vi "Create CAN Tag.vi"(8 "error in (no error)":errorcluster, 11 "CVT Tags to Create":T1) -> (0 "error out":errorcluster, 3 "CVT Tags to Create 2":T1)   [LabVIEW 2016, in "CVT.lvlib"]
uses:
  CVT.lvlib
  <vilib>/NI/Current Value Table/Type Defs/File Format.ctl
  <vilib>/NI/Current Value Table/Type Defs/Single Tag.ctl
  <vilib>/NI/Current Value Table/Type Defs/Data Types.ctl
  <vilib>/NI/Current Value Table/Type Defs/Tag Grouping set.ctl
  <vilib>/NI/Current Value Table/Current Value Table.lvlib
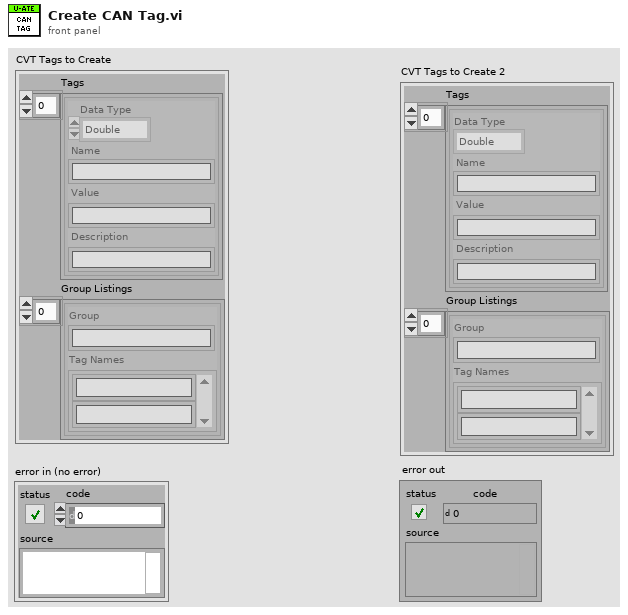
[diagram p1: front panel]
types:
  T1 = typedef "Current Value Table.lvlib/File Format.ctl" = cluster{"Tags":T2[], "Group Listings":T4[]}
  T2 = typedef "Current Value Table.lvlib/Single Tag.ctl" = cluster{"Data Type":T3, "Name":string, "Value":string, "Description":string}
  T3 = typedef "Current Value Table.lvlib/Data Types.ctl" = enum16{"Double", "Single", "I64", "I32", "I16", "I8", "U64", "U32", "U16", "U8", "String", "Boolean", "Array of U8", "Array of U16", "Array of U32", "Array of U64", "Array of I64", "Array of I32", "Array of I16", "Array of I8", "Array of Double", "Array of Single", "Array of Boolean", "Array of String"}
  T4 = typedef "Current Value Table.lvlib/Tag Grouping set.ctl" = cluster{"Group":string, "Tag Names":string[]}
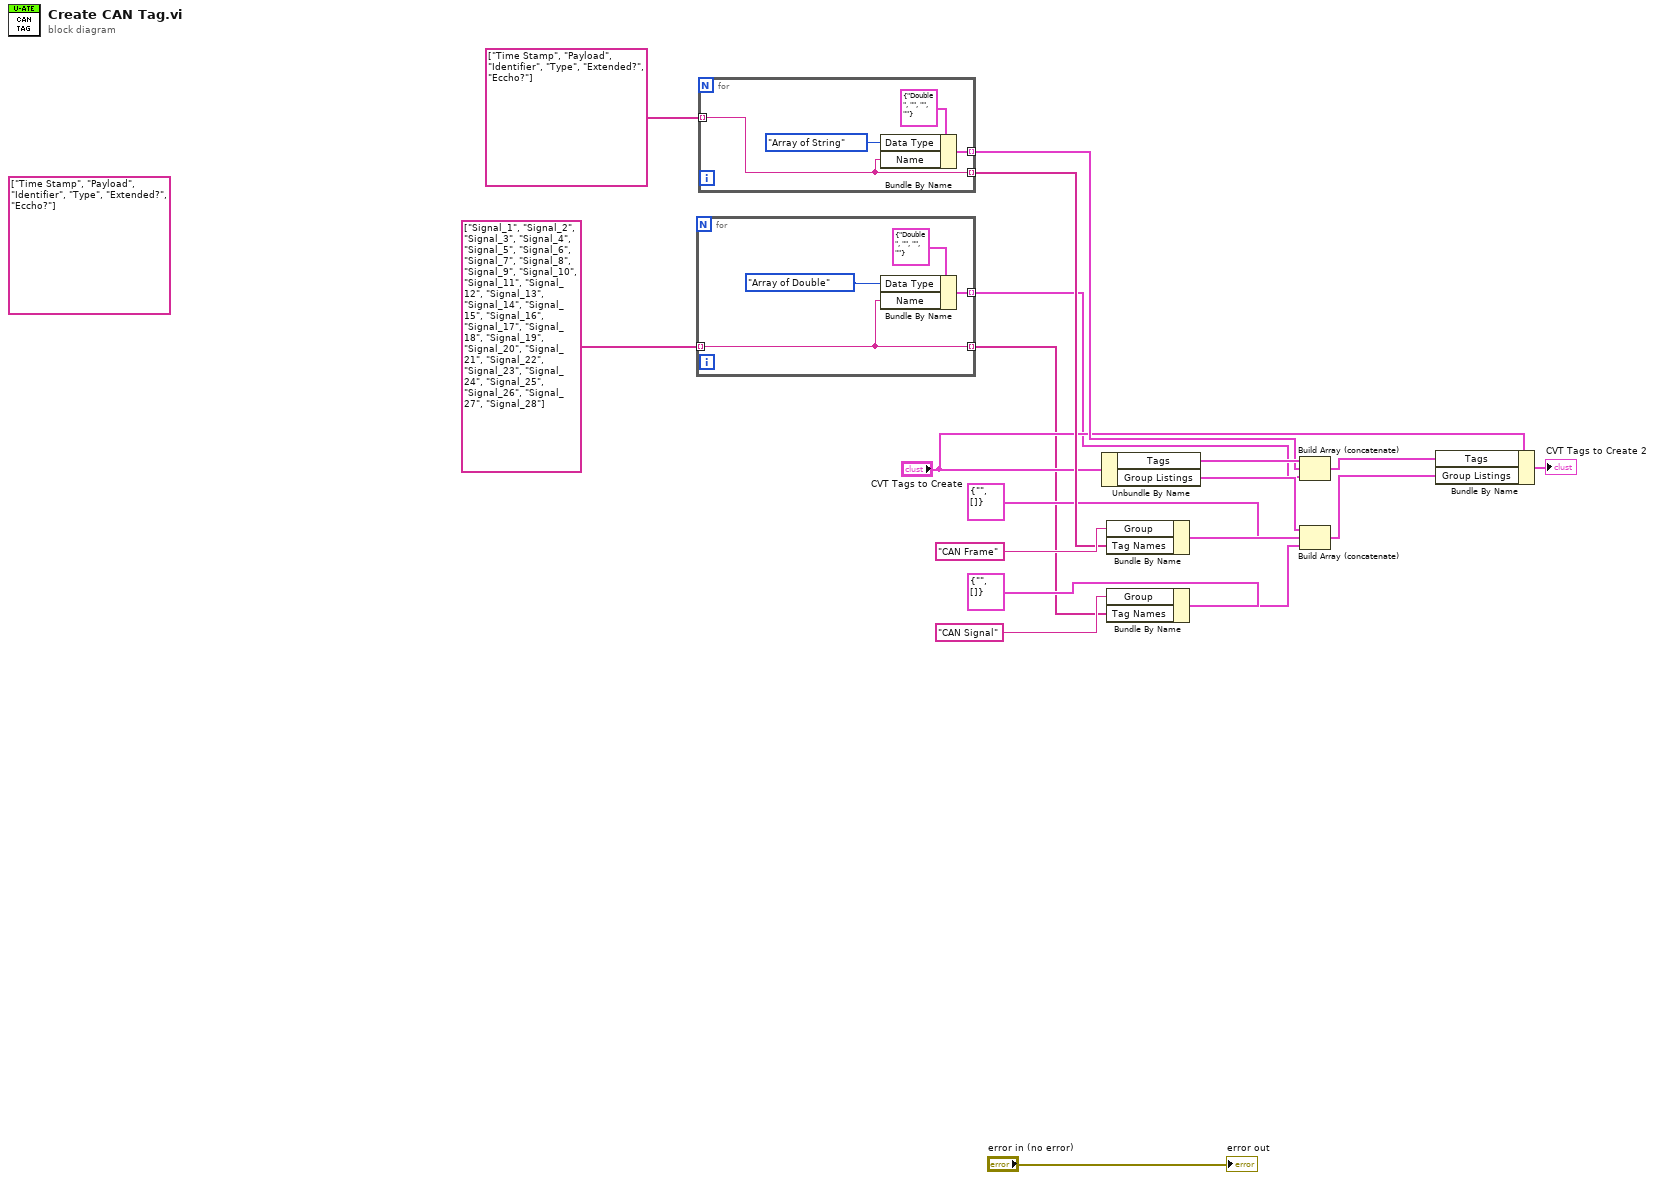
[diagram p0: block diagram]
diagram:
  (unwired) string[] ["Time Stamp", "Payload", "Identifier", "Type", "Extended?", "Eccho?"]
  n1 = for {
    tunnel: string[] ["Signal_1", "Signal_2", "Signal_3", "Signal_4", "Signal_5", "Signal_6", "Signal_7", "Signal_8", "Signal_9", "Signal_10", "Signal_11", "Signal_12", "Signal_13", "Signal_14", "Signal_15", "Signal_16", "Signal_17", "Signal_18", "Signal_19", "Signal_20", "Signal_21", "Signal_22", "Signal_23", "Signal_24", "Signal_25", "Signal_26", "Signal_27", "Signal_28"] ("Array 2") -> [w20] mode=indexing
    tunnel: [w21] -> w5 mode=indexing
    tunnel: [w20] -> w2 mode=indexing
    n2 = Bundle By Name(cluster=T2 {"Data Type"=enum."Double", "Name"="", "Value"="", "Description"=""} ("Tag"), "Data Type"=Data_Types."Array of Double", "Name"=w20) -> (w21:T2)
  }
  n3 = for {
    tunnel: string[] ["Time Stamp", "Payload", "Identifier", "Type", "Extended?", "Eccho?"] -> [w26] mode=indexing
    tunnel: [w27] -> w18 mode=indexing
    tunnel: [w26] -> w13 mode=indexing
    n4 = Bundle By Name(cluster=T2 {"Data Type"=enum."Double", "Name"="", "Value"="", "Description"=""} ("Tag"), "Data Type"=Data_Types."Array of String", "Name"=w26) -> (w27:T2)
  }
  n5 = Unbundle By Name("CVT Tags to Create") -> ("Tags"=w19:T2[], "Group Listings"=w12:T4[])
  n6 = Bundle By Name(cluster=T4 {"Group"="", "Tag Names"=[]} ("Tag Grouping"), "Group"="CAN Frame", "Tag Names"=w13) -> (w11:T4)
  n7 = Bundle By Name(cluster=T4 {"Group"="", "Tag Names"=[]} ("Tag Grouping"), "Group"="CAN Signal", "Tag Names"=w2) -> (w1:T4)
  n8 = Build Array (concatenate)(w19, w18, w5) -> (w17:T2[])
  n9 = Build Array (concatenate)(w12, w11, w1) -> (w10:T4[])
  n10 = Bundle By Name(cluster="CVT Tags to Create", "Tags"=w17, "Group Listings"=w10) -> (→"CVT Tags to Create 2":T1)
  "error out" <- "error in (no error)"
